vi "gRPC.Response.GetError.vi"(8 "error in (no error)":errorcluster, 11 "Response":variant) -> (0 "error out":errorcluster)   [LabVIEW 2025, in "XNET Bus Monitor Client.lvlib"]
uses:
  XNET Bus Monitor Client.lvlib
  xnet_can_bus_monitor_api_client/RPC Messages/ni_xnet_can_bm_api_ErrorInfo.ctl
  <userlib>/_OpenG.lib/lvdata/lvdata.llb/openg_variant.lvlib
  xnet_can_bus_monitor_api_client/xnet_can_bus_monitor_api_client.lvlib
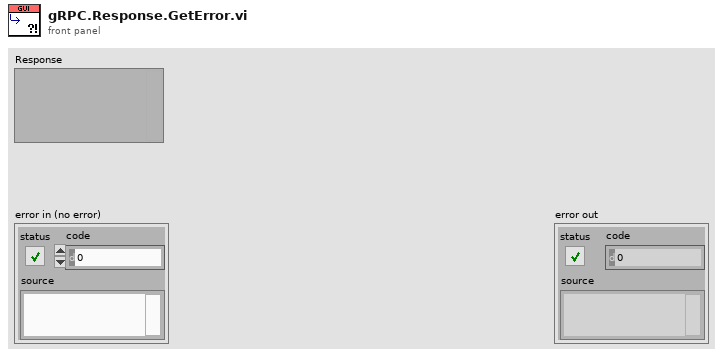
[diagram p1: front panel]
types:
  T1 = typedef "xnet_can_bus_monitor_api_client.lvlib/ni_xnet_can_bm_api_ErrorInfo.ctl" = errorcluster
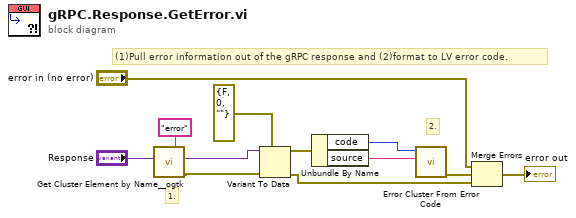
[diagram p0: block diagram]
diagram:
  # "2."
  # "1."
  # "(1)Pull error information out of the gRPC response and (2)format to LV error code."
  n1 = call <userlib>:"Get Cluster Element by Name__ogtk.vi"("Element Name"="error", "Cluster"="Response") -> ("error out"=w6:errorcluster, "VElement"=w5:variant)  [unwired: 7 in, 1 out]
  n2 = Variant To Data(error in=w6, type=T1 {"status"=FALSE, "code"=0, "source"=""} ("error"), Variant=w5) -> (data=w7:T1, error out=w12:errorcluster)
  n3 = Unbundle By Name(w7) -> ("code"=w9:i32, "source"=w10:string)
  n4 = call <vilib>:"Error Cluster From Error Code.vi"("error message (\"\")"=w10, "error code (0)"=w9) -> ("error out"=w8:errorcluster)  [unwired: 7 in]
  n5 = Merge Errors("error in (no error)", w8, w12) -> (→"error out":errorcluster)
